vi "read_params.vi"(8 "error in (no error)":errorcluster, 11 "AdaBoostRegressor in":refnum<class "AdaBoostRegressor.lvclass">) -> (0 "error out":errorcluster, 2 "params":T1={"base_estimator"="None", "n_estimators"=50.0, "learning_rate"=1.0, "loss"="linear", "random_state"=0.0}, 3 "AdaBoostRegressor out":refnum<class "AdaBoostRegressor.lvclass">)   [LabVIEW 2020, in "AdaBoostRegressor.lvclass"]
uses:
  AdaBoostRegressor.lvclass
  Controls/adaboostregressor_params.ctl
  AdaBoostRegressor.lvclass/AdaBoostRegressor.ctl
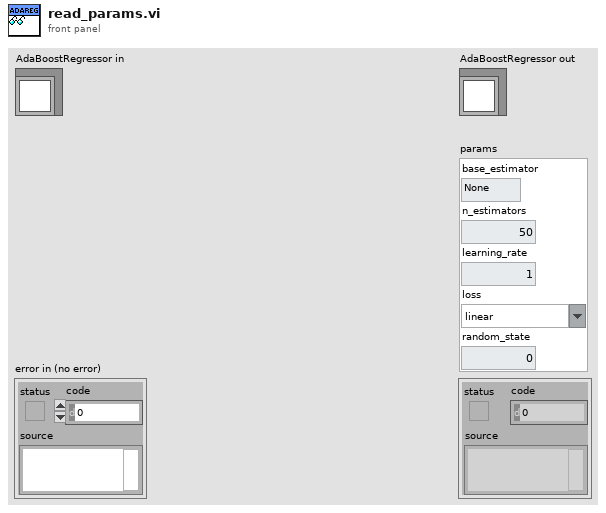
[diagram p1: front panel]
types:
  T1 = typedef "adaboostregressor_params.ctl" = cluster{"base_estimator":string, "n_estimators":dbl, "learning_rate":dbl, "loss":string, "random_state":dbl}
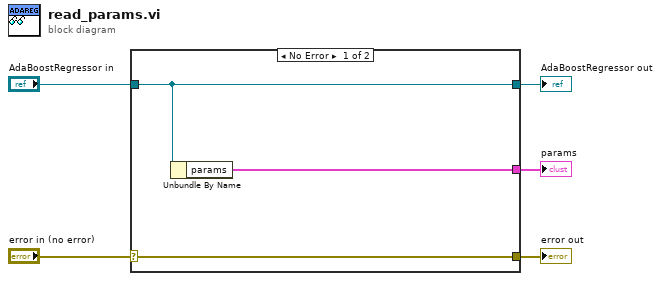
[diagram p0: block diagram]
diagram:
  n1 = case shown="No Error" "error in (no error)" {
    selector: "error in (no error)" -> [w8 w9]
    tunnel: [w8 w9] -> w4
    tunnel: [w7 w10] -> w2
    tunnel: "AdaBoostRegressor in" -> [w7 w10]
    tunnel: [w6 _] -> w1
    frame No Error {
      n2 = Unbundle By Name(w7) -> ("params"=w6:T1)
    }
    frame Error {
    }
  }
  "error out" <- w4
  "AdaBoostRegressor out" <- w2
  "params" <- w1
